vi "set gating.vi"(0 "2400 VISA":refnum<visa-resource-name>, 1 "gating type":T1=enum."2400", 3 "Source Measure Unit Channel (0: Channel A)":i32(ring) items=["Channel A", "Channel B"], 5 "2614 VISA":refnum<visa-resource-name>, 7 "Voltage Level":dbl, 9 "RATE(mV/s)":dbl format="%#_13g", 11 "error in (no error)":errorcluster, 12 "abort":refnum<vi>) -> (4 "VISA resource name out":refnum<visa-resource-name>, 15 "error out":errorcluster)   [LabVIEW 2019, in "SubVI.lvlib"]
uses:
  SubVI.lvlib
  ctl/Gating type.ctl
  User lib.lvlib
  lib/Keithley 2600 Series/Keithley 2600 Series.lvlib
panel:
  out "错误输出":errorcluster
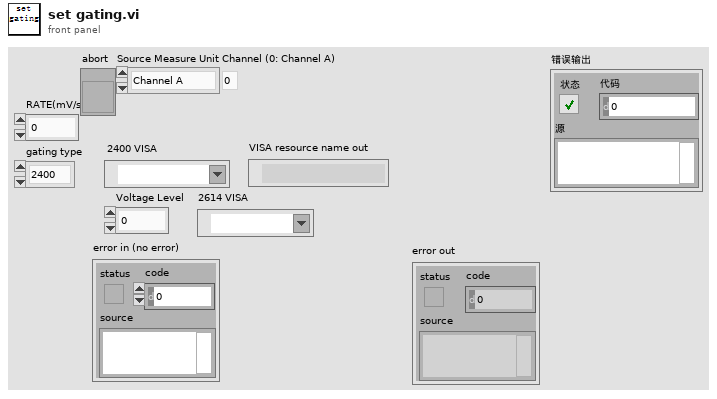
[diagram p1: front panel]
types:
  T1 = typedef "Gating type.ctl" = enum32{"null", "2614(daul)", "2400", "6517B"}
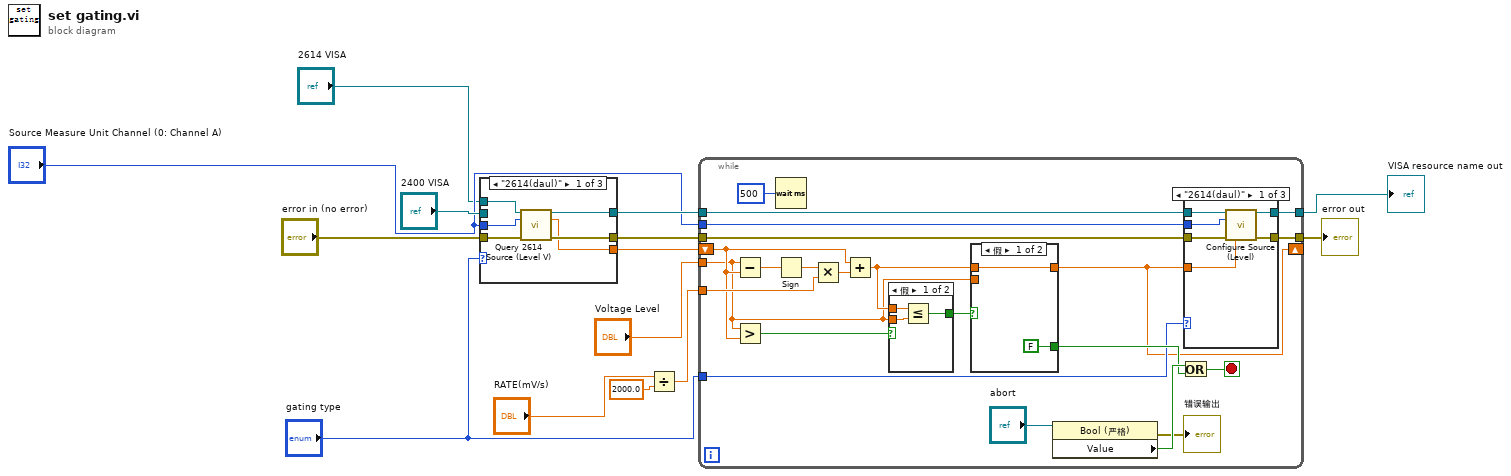
[diagram p0: block diagram]
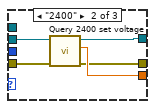
[diagram p2: hidden frame]
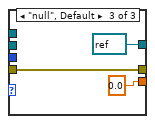
[diagram p3: hidden frame]
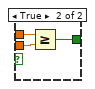
[diagram p4: hidden frame]
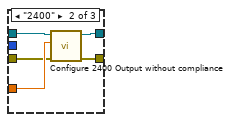
[diagram p5: hidden frame]
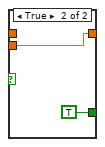
[diagram p7: hidden frame]
diagram:
  n1 = case shown="\"2614(daul)\"" "gating type" {
    tunnel: [w17 w25 0.0 ("Set Voltage")] -> w6
    tunnel: "2400 VISA" -> [_ w24 _]
    tunnel: [w19 w23 w28] -> w4
    tunnel: "error in (no error)" -> [w18 w22 w28]
    tunnel: [w20 w21 refnum<visa-resource-name> refnum ("VISA资源名称输出")] -> w3
    tunnel: "Source Measure Unit Channel (0: Channel A)" -> [w16 _ _]
    tunnel: "2614 VISA" -> [w15 _ _]
    frame "2614(daul)" {
      n2 = call "Query 2614 Source (Level V).vi"("VISA resource name"=w15, "Source Measure Unit Channel (0: Channel A)"=w16, "error in (no error)"=w18) -> ("VISA resource name out"=w20:refnum<visa-resource-name>, "levelv"=w17:dbl, "error out"=w19:errorcluster)  [unwired: 10 in]
    }
    frame "2400" {
      n3 = call "Query 2400 set voltage.vi"("错误输入（无错误）"=w22, "VISA资源名称"=w24) -> ("错误输出"=w23:errorcluster, "Set Voltage"=w25:dbl, "VISA资源名称输出"=w21:refnum<visa-resource-name>)  [unwired: 7 in]
    }
    frame "null", Default {
    }
  }
  n4 = Divide(x="RATE(mV/s)", y=2000.0) -> (x/y=w5:dbl)
  n5 = while {
    tunnel: w5 -> [w36]
    tunnel: "Voltage Level" -> [w30]
    tunnel: [w49] -> w12
    tunnel: w3 -> [w48]
    tunnel: [w43] -> w11
    tunnel: w4 -> [w41]
    tunnel: "Source Measure Unit Channel (0: Channel A)" -> [w40]
    tunnel: "gating type" -> [w39]
    shift-right: [w29] -> _
    shift-left: w6 -> [w34]
    stop <- w44 stop-if-true
    n6 = Subtract(x=w30, y=w34) -> (x-y=w38:dbl)
    n7 = Greater?(x=w30, y=w34) -> (0:w33:bool)
    n8 = Wait (ms)(milliseconds to wait=u32 500 ("等待时间（毫秒）")) -> ()  [unwired: 1 out]
    n9 = Sign(1:w38) -> (0:w37:dbl)
    n10 = Multiply(x=w37, y=w36) -> (x*y=w35:dbl)
    n11 = Add(x=w34, y=w35) -> (x+y=w32:dbl)
    n12 = case shown="假" w33 {
      tunnel: w30 -> [w52 w56]
      tunnel: w32 -> [w53 w55]
      tunnel: [w51 w54] -> w31
      frame False {
        n13 = Less Or Equal?(x=w53, y=w52) -> (x <= y?=w51:bool)
      }
      frame True {
        n14 = Greater Or Equal?(x=w55, y=w56) -> (x >= y?=w54:bool)
      }
    }
    n15 = case shown="假" w31 {
      tunnel: w32 -> [w71 _]
      tunnel: [w71 w72] -> w29
      tunnel: [FALSE TRUE] -> w45
      tunnel: w30 -> [_ w72]
      frame False {
      }
      frame True {
      }
    }
    n16 = property class="Bool (严格)"(reference="abort") -> (error out=→"错误输出":errorcluster, "Value"=w46:bool)  [unwired: 1 in, 1 out]
    n17 = Or(x=w46, y=w45) -> (x .or. y?=w44:bool)
    n18 = case shown="\"2614(daul)\"" w39 {
      tunnel: w29 -> [w57 w67 _]
      tunnel: [w62 w66 w69] -> w49
      tunnel: w48 -> [w59 w65 w69]
      tunnel: [w61 w64 w68] -> w43
      tunnel: w41 -> [w60 w63 w68]
      tunnel: w40 -> [w58 _ _]
      frame "2614(daul)" {
        n19 = call "Configure Source (Level).vi"("VISA resource name"=w59, "Source Measure Unit Channel (0: Channel A)"=w58, "error in (no error)"=w60, "Voltage Level (0 V)"=w57) -> ("VISA resource name out"=w62:refnum<visa-resource-name>, "error out"=w61:errorcluster)  [unwired: 10 in]
      }
      frame "2400" {
        n20 = call "Configure 2400 Output without compliance.vi"("error in (no error)"=w63, "Output Level (0)"=w67, "VISA resource name"=w65) -> ("error out"=w64:errorcluster, "VISA resource name out"=w66:refnum<visa-resource-name>)  [unwired: 7 in]
      }
      frame "null", Default {
      }
    }
  }
  "error out" <- w11
  "VISA resource name out" <- w12
